vi "Get Connection Information.vi"(8 "error in":errorcluster, 11 "instrument in":refnum<class "IInstrument.lvclass">) -> (0 "error out":errorcluster, 1 "port":u32, 2 "address":string, 3 "instrument out":refnum<class "IInstrument.lvclass">)   [LabVIEW 2020, in "MeasurementLink Session Management.lvlib" / "Session Reservation.lvclass"]
uses:
  Session Reservation.lvclass
  MeasurementLink Instrument/IInstrument/IInstrument.lvclass
  MeasurementLink Discovery Client/RPC Messages/ni_measurementlink_discovery_v1_ResolveServiceRequest.ctl
  MeasurementLink gRPC Utilities/TypeDefs/Service Location FGV Action.ctl
  Session Reservation.lvclass/Session Reservation.ctl
  MeasurementLink gRPC Utilities/MeasurementLink gRPC Utilities.lvlib
  MeasurementLink Discovery Client/MeasurementLink Discovery Client.lvlib
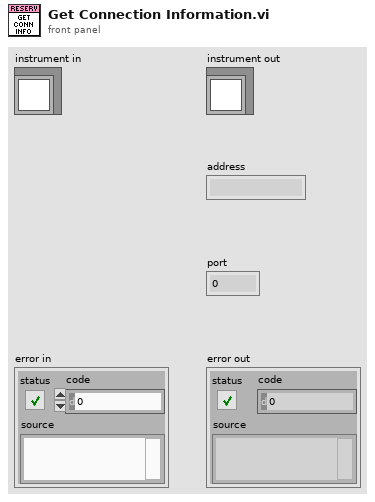
[diagram p1: front panel]
types:
  T1 = typedef "MeasurementLink Discovery Client.lvlib/ni_measurementlink_discovery_v1_ResolveServiceRequest.ctl" = cluster{"provided_interface":string, "service_class":string}
  T2 = typedef "MeasurementLink gRPC Utilities.lvlib/Service Location FGV Action.ctl" = enum16{"Get Service Location", "Clear Cache"}
  T3 = typedef "MeasurementLink Discovery Client.lvlib/ni_measurementlink_discovery_v1_ServiceLocation.ctl" = cluster{"location":string, "insecure_port":string, "ssl_authenticated_port":string}
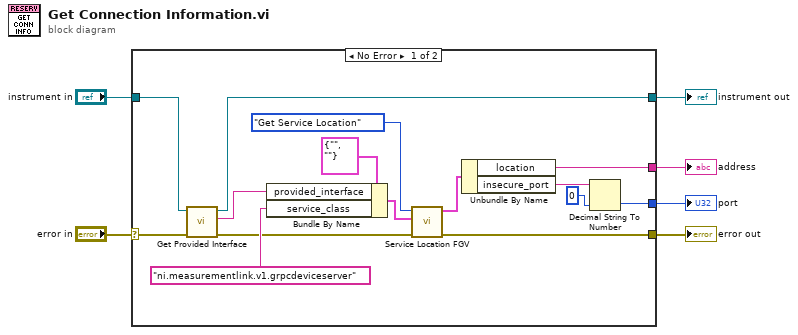
[diagram p0: block diagram]
diagram:
  n1 = case shown="No Error" "error in" {
    selector: "error in" -> [w7 w23]
    tunnel: [w19 _] -> w6
    tunnel: [w18 _] -> w5
    tunnel: [w16 w23] -> w4
    tunnel: [w10 w22] -> w3
    tunnel: "instrument in" -> [w8 w22]
    frame No Error {
      n2 = call-dynamic "Get Provided Interface.vi"("error in (no error)"=w7, "instrument in"=w8) -> ("error out"=w9:errorcluster, "provided interface"=w14:string, "instrument out"=w10:refnum<class "IInstrument.lvclass">)  [unwired: 7 in]
      n3 = Bundle By Name(cluster=T1 {"provided_interface"="", "service_class"=""} ("Resolve Service Request"), "provided_interface"=w14, "service_class"="ni.measurementlink.v1.grpcdeviceserver") -> (w11:T1)
      n4 = call "Service Location FGV.vi"("error in"=w9, "Resolve Service Request"=w11, "Action"=Service_Location_FGV_Action."Get Service Location") -> ("error out"=w16:errorcluster, "Service Location"=w20:T3)  [unwired: 7 in]
      n5 = Unbundle By Name(w20) -> ("location"=w18:string, "insecure_port"=w17:string)
      n6 = Decimal String To Number(string=w17, default (0L)=u32 0 ("default (0 I32)")) -> (number=w19:u32)  [unwired: 1 in, 1 out]
    }
    frame Error {
    }
  }
  "port" <- w6
  "address" <- w5
  "error out" <- w4
  "instrument out" <- w3
